vi "Write Text labels.vi"(5 "Text labels":string[](array[string]), 9 "NumericWithScale in":refnum<class "NumericWithScale.lvclass">) -> (3 "NumericWithScale out":refnum<class "NumericWithScale.lvclass">)   [LabVIEW 2014, in "NumericWithScale.lvclass"]
uses:
  NumericWithScale.lvclass
  NumericWithScale.lvclass/NumericWithScale.ctl
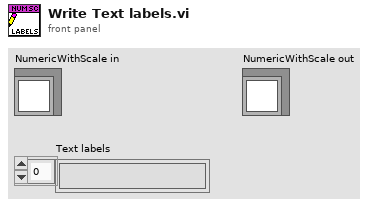
[diagram p1: front panel]
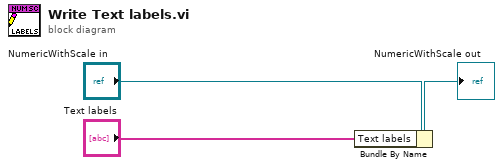
[diagram p0: block diagram]
diagram:
  n1 = Bundle By Name(cluster="NumericWithScale in", "Text labels"="Text labels") -> (→"NumericWithScale out":refnum<class "NumericWithScale.lvclass">)
